vi "Scan End Mode.vi"(7 "Read Value? (F)":bool, 8 "error in (no error)":errorcluster, 10 "Scan End Mode (Stop)":T1, 11 "VISA resource name":refnum<visa-resource-name>) -> (0 "error out":errorcluster, 2 "Scan End Mode":T1, 3 "VISA resource name out":refnum<visa-resource-name>)   [LabVIEW 2013, in "SRS SR400.lvlib"]
doc: "<B>NE { j }</B>\n\nIf j = 0, the NE command sets the scan end mode (AT N) to STOP. If j = 1, the mode is set to START. The scan end mode may be changed at any time. If j is absent, the scan end mode is returned."
uses:
  <instrlib>/SRS SR400/SRS SR400.lvlib
  <instrlib>/SRS SR400/Public/Typedefs/Scan End Mode.ctl
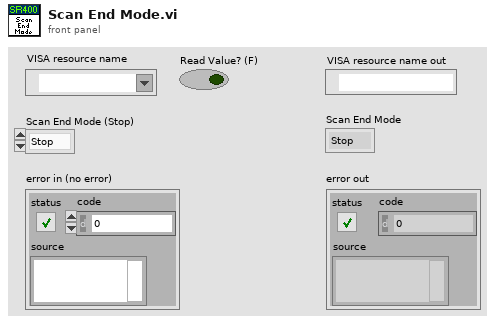
[diagram p1: front panel]
types:
  T1 = typedef "SRS SR400.lvlib/Scan End Mode.ctl" = enum16{"Stop", "Start"}
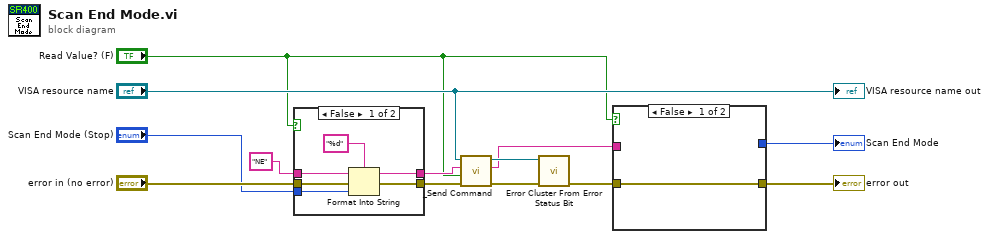
[diagram p0: block diagram]
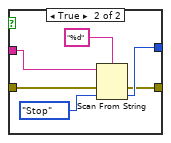
[diagram p2: hidden frame]
diagram:
  n1 = case shown="False" "Read Value? (F)" {
    tunnel: "error in (no error)" -> [w19 w20]
    tunnel: "NE" ("command") -> [w17 w21]
    tunnel: [w16 w21] -> w11
    tunnel: [w15 w20] -> w10
    tunnel: "Scan End Mode (Stop)" -> [w14 _]
    frame False {
      n2 = Format Into String(format string="%d", initial string=w17, error in=w19, w14) -> (resulting string=w16:string, error out=w15:errorcluster)
    }
    frame True {
    }
  }
  n3 = call <instrlib>:"_Send Command.vi"("error in (no error)"=w10, "Read Value? (F)"="Read Value? (F)", "Command"=w11, "VISA resource name"="VISA resource name") -> ("error out"=w6:errorcluster, "Response"=w4:string, "VISA resource name out"=w7:refnum<visa-resource-name>)  [unwired: 5 out]
  n4 = call <instrlib>:"Error Cluster From Error Status Bit.vi"("error in (no error)"=w6, "VISA resource name"=w7) -> ("error out"=w5:errorcluster)  [unwired: 8 in, 1 out]
  n5 = case shown="False" "Read Value? (F)" {
    tunnel: w5 -> [w22 w28]
    tunnel: w4 -> [_ w26]
    tunnel: [_ w24] -> w2
    tunnel: [w22 w23] -> w1
    frame False {
    }
    frame True {
      n6 = Scan From String(format string="%d", input string=w26, error in=w28, default 1=Scan_End_Mode."Stop" ("Scan End Mode (Stop)")) -> (error out=w23:errorcluster, output 1=w24:T1)  [unwired: 1 in, 2 out]
    }
  }
  "error out" <- w1
  "Scan End Mode" <- w2
  "VISA resource name out" <- "VISA resource name"
